vi "Queue_Comm_FGV.vi"(8 "error in (no error)":errorcluster, 10 "Enum":T1, 11 "queue in":refnum<queue>) -> (0 "error Out":errorcluster, 3 "queue Out":refnum<queue>)   [LabVIEW 2024, in "PCANusb_DTU.lvlib"]
doc: "This VI\n-----------------------------------\nQueue_Comm_FGV\n-----------------------------------\n-Craetes a FG varaibale for queue reference"
uses:
  PCANusb_DTU.lvlib
  PrivateControls/FGV_Queue_Control.ctl
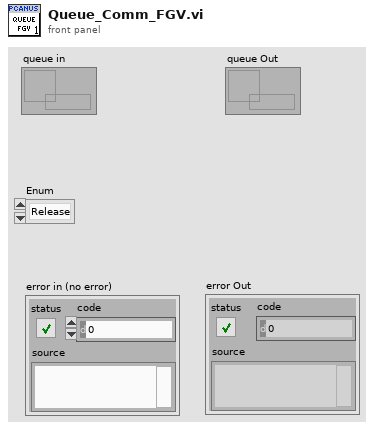
[diagram p1: front panel]
types:
  T1 = typedef "PCANusb_DTU.lvlib/FGV_Queue_Control.ctl" = enum16{"Release", "Flush", "Get", "Set"}
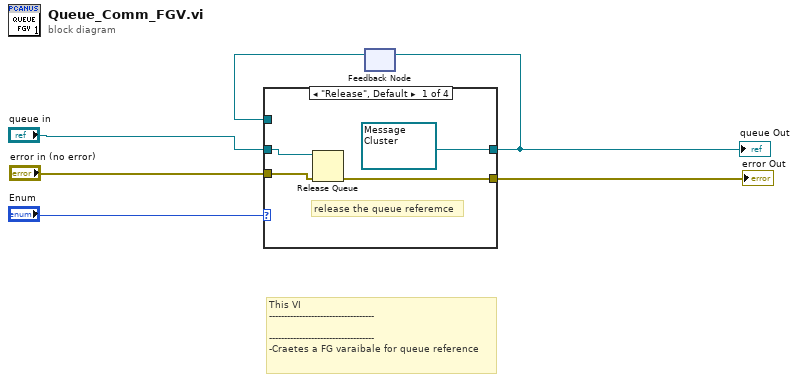
[diagram p0: block diagram]
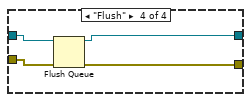
[diagram p4: hidden frame]
diagram:
  # "This VI\n-----------------------------------\n\n-----------------------------------\n-Craetes a FG varaibale for queue reference"
  n1 = feedback #1() -> (w5:refnum<queue>)  [unwired: 1 in]
  n2 = case shown="\"Release\", Default" "Enum" {
    tunnel: "queue in" -> [w7 _ w14 w15]
    tunnel: [refnum<queue> refnum ("queue out") w12 w14 w16] -> w1
    tunnel: w5 -> [_ w12 _ _]
    tunnel: "error in (no error)" -> [w10 w11 w13 w18]
    tunnel: [w9 w11 w13 w17] -> w3
    frame "Release", Default {
      # "release the queue referemce"
      n3 = Release Queue(queue=w7, error in (no error)=w10) -> (error out=w9:errorcluster)  [unwired: 1 in, 2 out]
    }
    frame "Get" {
      # "get  the queue reference in FGV"
    }
    frame "Set" {
      # "set the queue reference in FGV"
    }
    frame "Flush" {
      n4 = Flush Queue(queue=w15, error in (no error)=w18) -> (queue out=w16:refnum<queue>, error out=w17:errorcluster)  [unwired: 1 out]
    }
  }
  "error Out" <- w3
  "queue Out" <- w1
  n5 = feedback-in #1(w1) -> ()
